vi "Button Invoke.vi"(10 "VI Refnum in":refnum<vi>, 11 "Boolean in":refnum<vi>) -> (3 "VI out":refnum<vi>)   [LabVIEW 2014]
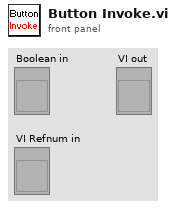
[diagram p1: front panel]
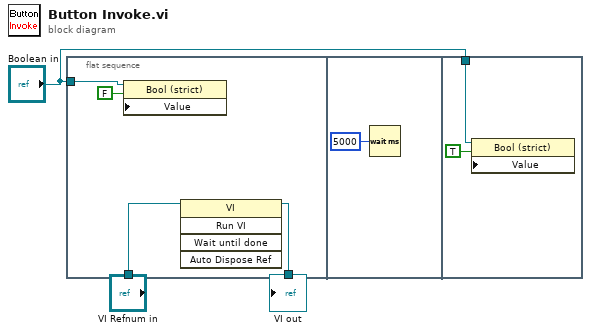
[diagram p0: block diagram]
diagram:
  n1 = flat-sequence {
    tunnel: "VI Refnum in" -> [w6]
    tunnel: [w5] -> w3
    tunnel: "Boolean in" -> [w4]
    tunnel: "Boolean in" -> [w9]
    frame #0 {
      n2 = property class="Bool (strict)"(reference=w4, "Value"=FALSE ("Right Continuer")) -> ()  [unwired: 1 in, 2 out]
      n3 = invoke class="VI" method="Run VI"(reference=w6) -> (reference out=w5:refnum<vi>)  [unwired: 4 in, 4 out]
    }
    frame #1 {
      n4 = Wait (ms)(milliseconds to wait=u32 5000) -> ()  [unwired: 1 out]
    }
    frame #2 {
      n5 = property class="Bool (strict)"(reference=w9, "Value"=TRUE ("Right Continuer")) -> ()  [unwired: 1 in, 2 out]
    }
  }
  "VI out" <- w3
